vi "输出控制.vi"(8 "输入读取输入":T5) -> (3 "输出控制输出":T1)   [LabVIEW 2017]
panel:
  in  "选项卡控件":enum32{"选项卡 1", "选项卡 2"}(tab)
  out "运行时间":dbl
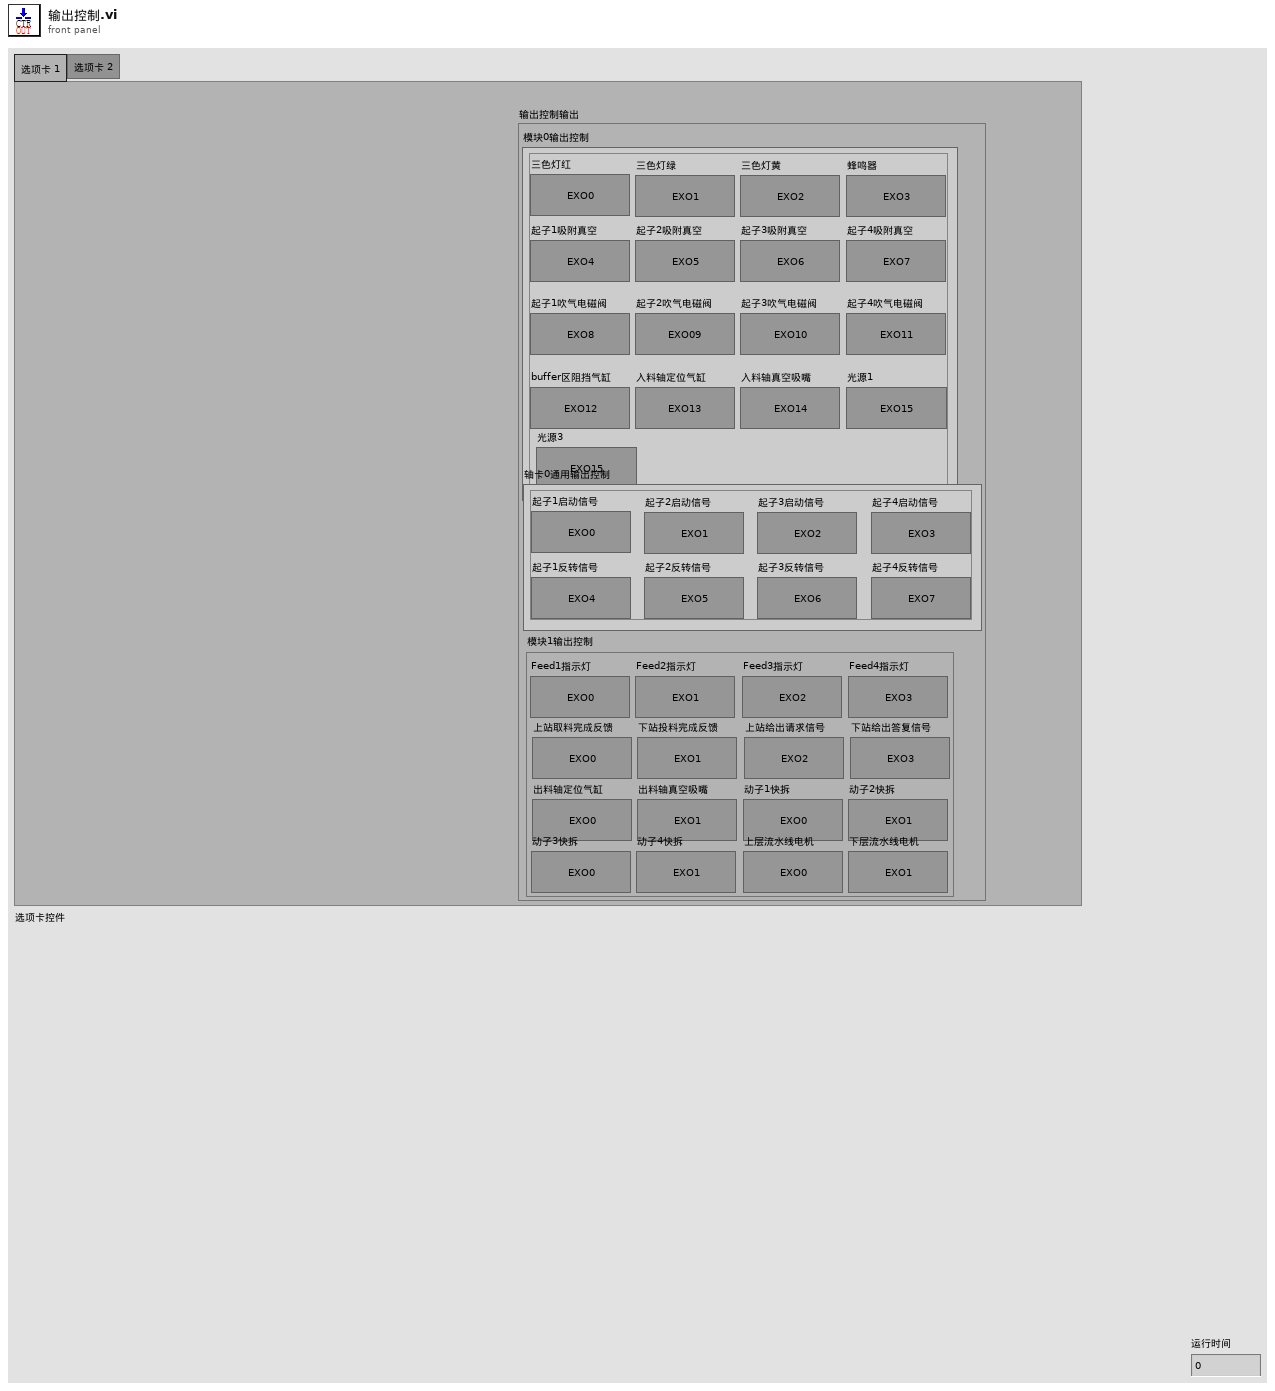
[diagram p1: front panel]
types:
  T1 = typedef "输出控制.ctl" = cluster{"模块0输出控制":T2, "轴卡0通用输出控制":T3, "模块1输出控制":T4}
  T2 = typedef "模块0输出控制.ctl" = cluster{"三色灯红":bool, "三色灯绿":bool, "三色灯黄":bool, "蜂鸣器":bool, "起子1吸附真空":bool, "起子2吸附真空":bool, "起子3吸附真空":bool, "起子4吸附真空":bool, "起子1吹气电磁阀":bool, "起子2吹气电磁阀":bool, "起子3吹气电磁阀":bool, "起子4吹气电磁阀":bool, "buffer区阻挡气缸":bool, "入料轴定位气缸":bool, "入料轴真空吸嘴":bool, "光源1":bool, "光源3":bool}
  T3 = typedef "轴卡0通用输出控制.ctl" = cluster{"起子1启动信号":bool, "起子2启动信号":bool, "起子3启动信号":bool, "起子4启动信号":bool, "起子1反转信号":bool, "起子2反转信号":bool, "起子3反转信号":bool, "起子4反转信号":bool}
  T4 = typedef "模块1输出控制.ctl" = cluster{"Feed1指示灯":bool, "Feed2指示灯":bool, "Feed3指示灯":bool, "Feed4指示灯":bool, "上站取料完成反馈":bool, "下站投料完成反馈":bool, "上站给出请求信号":bool, "下站给出答复信号":bool, "出料轴定位气缸":bool, "出料轴真空吸嘴":bool, "动子1快拆":bool, "动子2快拆":bool, "动子3快拆":bool, "动子4快拆":bool, "上层流水线电机":bool, "下层流水线电机":bool}
  T5 = typedef "输入读取.ctl" = cluster{"模块0输入信号":T6, "轴卡通用输入读取":T7, "模块1输入信号":T8, "轴卡1通用输入读取":T9}
  T6 = typedef "模块0输入读取.ctl" = cluster{"启动按钮":bool, "复位按钮":bool, "暂停按钮":bool, "操作侧安全光栅":bool, "后侧安全光栅":bool, "起子1真空检知":bool, "起子2真空检知":bool, "起子3真空检知":bool, "起子4真空检知":bool, "feed01感应sensor":bool, "feed02感应sensor":bool, "feed03感应sensor":bool, "feed04感应sensor":bool, "阻挡气缸前位":bool, "阻挡气缸后位":bool, "buffer1感应sensor":bool}
  T7 = typedef "轴卡0通用输入读取.ctl" = cluster{"buffer2感应sensor1":bool, "buffer2感应sensor2":bool, "入料轴定位气缸前位":bool, "入料轴定位气缸后位":bool, "入料轴定位sensor1":bool, "入料轴定位sensor2":bool, "入料轴真空检知":bool, "出料轴定位气缸前位":bool, "出料轴定位气缸后位":bool, "出料轴定位sensor1":bool, "上站允许取料信号":bool, "下站允许投料信号":bool, "起子1扭力达到信号":bool, "起子2扭力达到信号":bool, "起子3扭力达到信号":bool, "起子4扭力达到信号":bool}
  T8 = typedef "模块1输入读取.ctl" = cluster{"出料轴定位sensor2":bool, "出料轴真空检知":bool, "出入料交互感应1":bool, "出入料交互感应2":bool}
  T9 = typedef "轴卡1通用输入读取.ctl" = cluster{"上站请求信号":bool, "下站答复信号":bool, "起子1ready信号":bool, "起子2ready信号":bool, "起子3ready信号":bool, "起子4ready信号":bool, "出料区感应sensor":bool, "安全光栅1":bool, "安全光栅2":bool}
  T10 = typedef "MX操作选项.ctl" = enum16{"MX Initial ", "MX Close", "X&Y&M Read", "X&Y&M Write", "D Read", "D Write", "Many component Read", "Many component Write", "Load Function Global"}
  T11 = typedef "Component Assemble Input.ctl" = cluster{"Component Name":string, "Component State":bool, "D Value":i32}
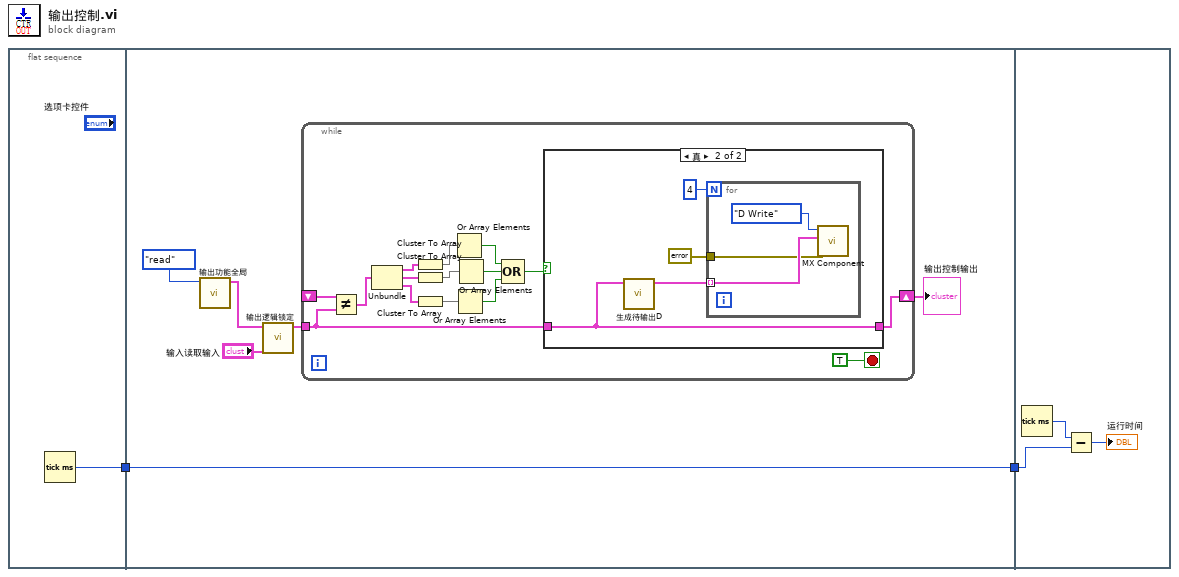
[diagram p0: block diagram]
diagram:
  n1 = flat-sequence {
    tunnel: [w3] -> w2
    tunnel: w2 -> [w9]
    tunnel: [w9] -> w1
    tunnel: w1 -> [w34]
    frame #0 {
      n2 = Tick Count (ms)() -> (millisecond timer value=w3:u32)
    }
    frame #1 {
      n3 = call "输出功能全局.vi"("选项"=enum16{"initialize", "read", "write"}."read") -> ("输出控制"=w4:T1)  [unwired: 10 in]
      n4 = call "输出逻辑锁定.vi"("输入读取输入"="输入读取输入", "输出控制"=w4) -> ("输出控制输出"=w8:T1)  [unwired: 9 in]
      n5 = while {
        shift-right: [w23] -> w7
        shift-left: _ -> [w22]
        tunnel: w8 -> [w21]
        stop <- TRUE stop-if-true
        n6 = Not Equal?(x=w22, y=w21) -> (x != y?=w20:T1)
        n7 = Unbundle(w20) -> ("模块0输出控制"=w19:T2, "轴卡0通用输出控制"=w18:T3, "模块1输出控制"=w17:T4)
        n8 = Cluster To Array(cluster=w19) -> (array=w16:bool[])
        n9 = Cluster To Array(cluster=w18) -> (array=w14:bool[])
        n10 = Cluster To Array(cluster=w17) -> (array=w15:bool[])
        n11 = Or Array Elements(Boolean array=w16) -> (logical OR=w13:bool)
        n12 = Or Array Elements(Boolean array=w15) -> (logical OR=w11:bool)
        n13 = Or Array Elements(Boolean array=w14) -> (logical OR=w12:bool)
        n14 = Compound Arithmetic op=OR(w13, w12, w11) -> (w10:bool)
        n15 = case shown="真" w10 {
          tunnel: w21 -> [w25 w27]
          tunnel: [w25 w27] -> w23
          frame False {
          }
          frame True {
            n16 = call "生成待输出D.vi"("输出控制"=w27) -> ("待输出操作"=w26:T11[])  [unwired: 10 in]
            n17 = for {
              N: 4 -> [_]
              tunnel: w26 -> [w31] mode=indexing
              tunnel: errorcluster {"status"=FALSE, "code"=0, "source"=""} ("错误输入") -> [w30]
              n18 = call "MX Component.vi"("错误输入"=w30, "Component Assemble Input"=w31, "MX操作选项"=MX操作选项."D Write") -> ()  [unwired: 7 in, 2 out]
            }
          }
        }
      }
      "输出控制输出" <- w7
    }
    frame #2 {
      n19 = Tick Count (ms)() -> (millisecond timer value=w35:u32)
      n20 = Subtract(x=w35, y=w34) -> (x-y=→"运行时间":u32)
    }
  }
